vi "Find Files and Replace With 0 and 1 array.vi"(10 "regular expression":string, 11 "filenames":string[](array[string])) -> (3 "Array":string[](array[string]))   [LabVIEW 2012]
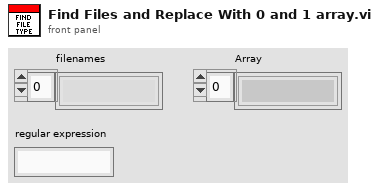
[diagram p1: front panel]
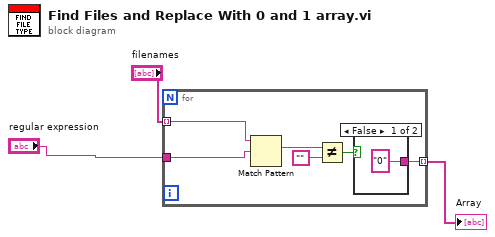
[diagram p0: block diagram]
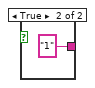
[diagram p2: hidden frame]
diagram:
  n1 = for {
    tunnel: "filenames" -> [w9] mode=indexing
    tunnel: [w5] -> w1 mode=indexing
    tunnel: "regular expression" -> [w4]
    n2 = Match Pattern(string=w9, regular expression=w4) -> (match substring=w8:string)  [unwired: 1 in, 3 out]
    n3 = Not Equal?(x=w8, y="") -> (x != y?=w6:bool)
    n4 = case shown="False" w6 {
      tunnel: ["0" "1"] -> w5
      frame False {
      }
      frame True {
      }
    }
  }
  "Array" <- w1
